vi "Combine Device Info.vi"(8 "error in (no error)":errorcluster, 10 "DeviceInfo":string, 11 "Device in":refnum<class "Device.lvclass">) -> (0 "error out":errorcluster, 1 "Combined Device":string, 2 "Device Code":string, 3 "Device out":refnum<class "Device.lvclass">, 4 "Bit Device?":bool)   [LabVIEW 2019, in "SLMP.lvlib" / "Device.lvclass"]
uses:
  Device.lvclass
  Device.lvclass/Device.ctl
  8d35433b-f5a1-4041-a90d-80a323363962.vi
  <vilib>/JDP Science/JSONtext/String Subset.vi
  <vilib>/JDP Science/JSONtext/Parsing/Parse Full Path or Item Name.vi
  <vilib>/JDP Science/JSONtext/Next JSON Value.vi
  <vilib>/JDP Science/JSONtext/support/Error Cluster From Code.vi
  <vilib>/JDP Science/JSONtext/Offset/Find Item Locations by Path.vi
  <vilib>/JDP Science/JSONtext/Set Multiple Object Items.vi
  <vilib>/JDP Science/JSONtext/JSON text to Variant.vi
  <vilib>/JDP Science/JSONtext/LVClass Serializer/JSONtext LVClass Serializer.lvclass
  <vilib>/JDP Science/JSONtext/JSONtext.lvlib
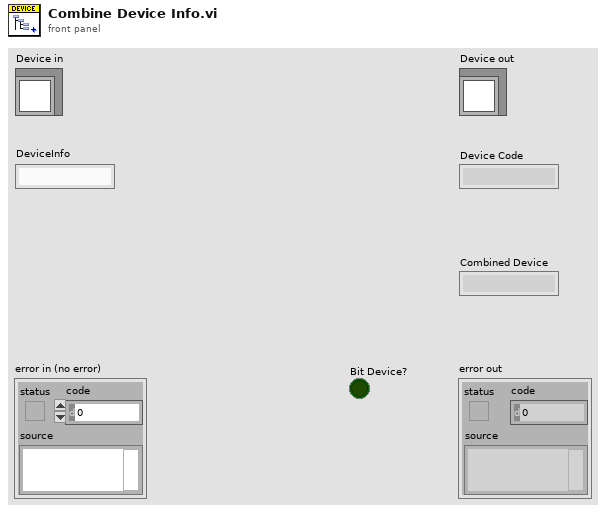
[diagram p1: front panel]
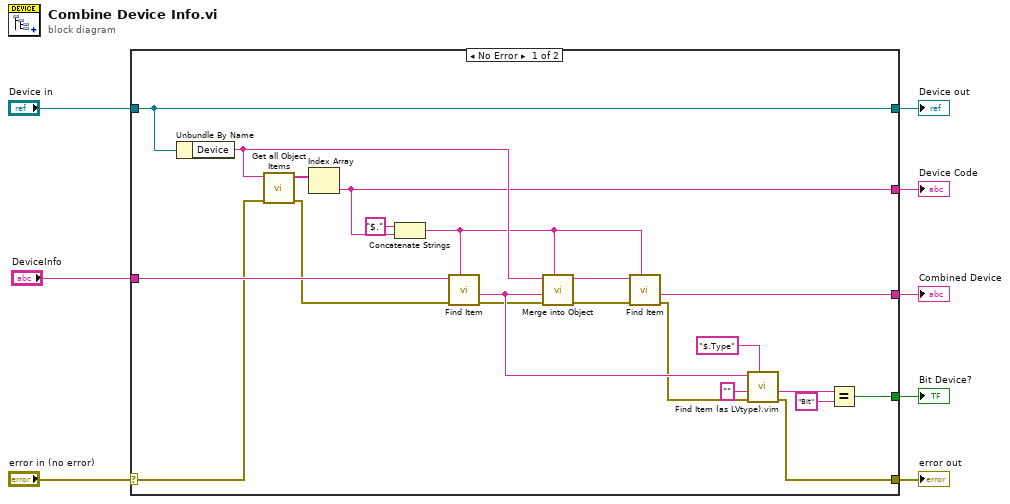
[diagram p0: block diagram]
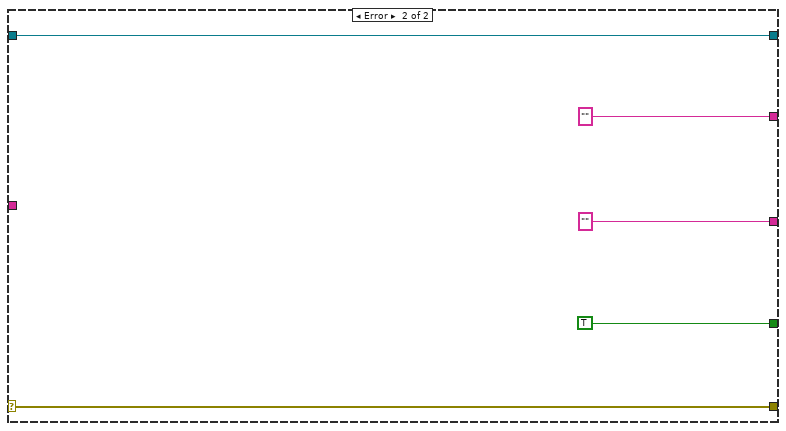
[diagram p2: hidden frame]
diagram:
  n1 = case shown="No Error" "error in (no error)" {
    selector: "error in (no error)" -> [w10 w34]
    tunnel: [w11 w34] -> w7
    tunnel: [w29 w33] -> w5
    tunnel: "Device in" -> [w29 w33]
    tunnel: "DeviceInfo" -> [w27 _]
    tunnel: [w15 "" ("<JSON>")] -> w3
    tunnel: [w19 TRUE] -> w2
    tunnel: [w18 "" ("substring")] -> w1
    frame No Error {
      n2 = Unbundle By Name(w29) -> ("Device"=w25:string)
      n3 = call <vilib>:"Get all Object Items.vi"("error in (no error)"=w10, "JSON"=w25) -> ("error out"=w9:errorcluster, "Item Names"=w28:string[])  [unwired: 6 in, 2 out]
      n4 = Index Array(array=w28) -> (element=w18:string)  [unwired: 1 in]
      n5 = Concatenate Strings("$." ("string"), w18) -> (w14:string)
      n6 = call <vilib>:"Find Item.vi"("$Path or Item Name"=w14, "error in (no error)"=w9, "JSON"=w27) -> ("error out"=w13:errorcluster, "<JSON>"=w24:string)  [unwired: 5 in, 2 out]
      n7 = call <vilib>:"Merge into Object.vi"("$Path or Item Name"=w14, "error in (no error)"=w13, "JSON Object to Merge"=w24, "JSON"=w25) -> ("error out"=w16:errorcluster, "<JSON>"=w17:string)  [unwired: 5 in]
      n8 = call <vilib>:"Find Item.vi"("$Path or Item Name"=w14, "error in (no error)"=w16, "JSON"=w17) -> ("error out"=w12:errorcluster, "<JSON>"=w15:string)  [unwired: 5 in, 2 out]
      n9 = call "Find Item (as LVtype).vim"("$Path or Item Name"="$.Type", "error in (no error)"=w12, "Data Type and Default Value"="", "JSON"=w24) -> ("error out"=w11:errorcluster, "Data"=w21:string)  [unwired: 4 in, 2 out]
      n10 = Equal?(x=w21, y="Bit") -> (x = y?=w19:bool)
    }
    frame Error {
    }
  }
  "error out" <- w7
  "Device out" <- w5
  "Combined Device" <- w3
  "Bit Device?" <- w2
  "Device Code" <- w1
